vi "7HP_Get_ax_ay_az.vi"(6 "7HP Name":string, 9 "Time Trace":T1[](array[typedef]), 10 "Analysis Info cluster":T2[](array[typedef]) {"Sync Delay Time (s)" format="%.4f"; "Sd Error in Variance" format="%.2f"; "Skew_u" format="%.2f"; "% u'/U" format="%.2f"; "Sd Error in Mean" format="%.2f"; "Kurt_u" format="%.2f"; "u^4" format="%.2f"; "u^3" format="%.2f"; "U" format="%.2f"; "u^2" format="%.2f"}, 11 "Pressure Index":i32[](array[numeric])) -> (3 "ax ay az":sgl[](array[numeric]))   [LabVIEW 2018]
uses:
  Controls/Analysis_info_cluster.ctl
  Controls/Inst_type.ctl
  Controls/Instrument_Array.ctl
  Controls/Time_Trace_Cluster.ctl
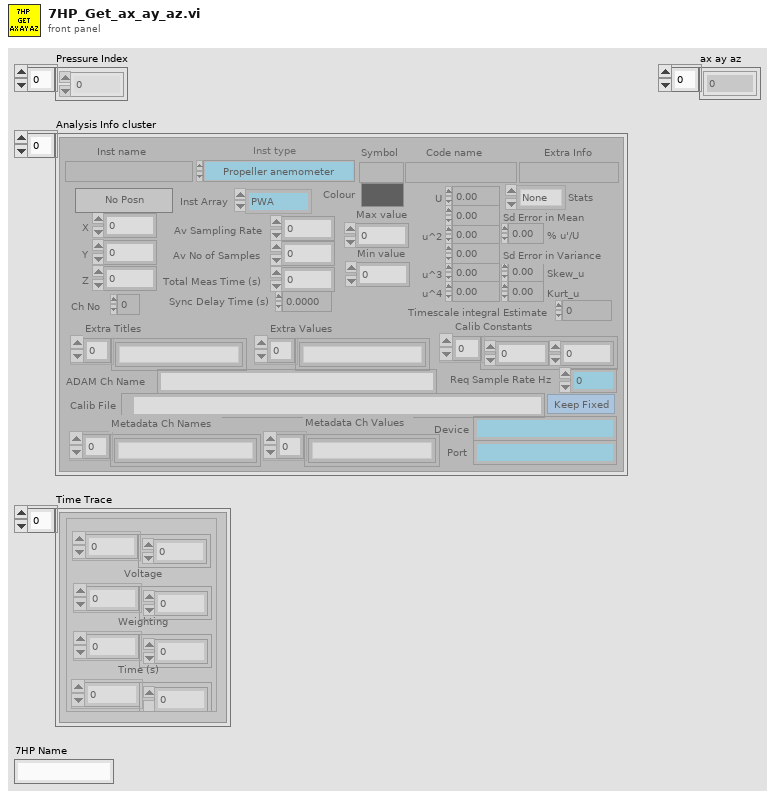
[diagram p1: front panel]
types:
  T1 = typedef "Time_Trace_Cluster.ctl" = cluster{"Weighting":dbl[], "Time (s)":dbl[], "Voltage":dbl[], "Eng Values":dbl[]}
  T2 = typedef "Analysis_info_cluster.ctl" = cluster{"Colour":u32, "Inst type":T3, "Inst name":string, "Symbol":string, "Code name":string, "Extra Info":string, "Inst Array":T4, "Extra Titles":string[], "Extra Values":string[], "U":dbl, "u^2":dbl, "u^3":dbl, "u^4":dbl, "Skew_u":dbl, "Kurt_u":dbl, "Sd Error in Mean":dbl, "% u'/U":dbl, "X":dbl, "Y":dbl, "Z":dbl, "Timescale integral Estimate":dbl, "Sd Error in Variance":dbl, "Calib File":path, "Calib Constants":dbl[], "Output Position":bool, "Stats":enum16{"None", "Basic", "Full"}, "Av Sampling Rate":dbl, "Av No of Samples":dbl, "Total Meas Time (s)":dbl, "ADAM Ch Name":string, "Max value":dbl, "Min value":dbl, "Req Sample Rate Hz":dbl, "Sync Delay Time (s)":dbl, "Ch No":i16, "Device":string, "Use Latest Calib":bool, "Port":string, "Metadata Ch Names":string[], "Metadata Ch Values":string[]}
  T3 = typedef "Inst_type.ctl" = enum16{"Propeller anemometer", "Raw voltage", "Pressure Transducer", "Pitot-static tube", "Preston tube", "Hot wire", "Cross wire 1", "Cross wire 2", "Generic Linear", "Generic Polynomial", "Generic BackPoly", "Fast FID", "Thermocouple", "Cold wire", "Pulsed Wire", "LDA Vel", "LDA Tran time", "LDA Arr time", "Microphone"}
  T4 = typedef "Instrument_Array.ctl" = enum16{"PWA", "LDA", "Analogue"}
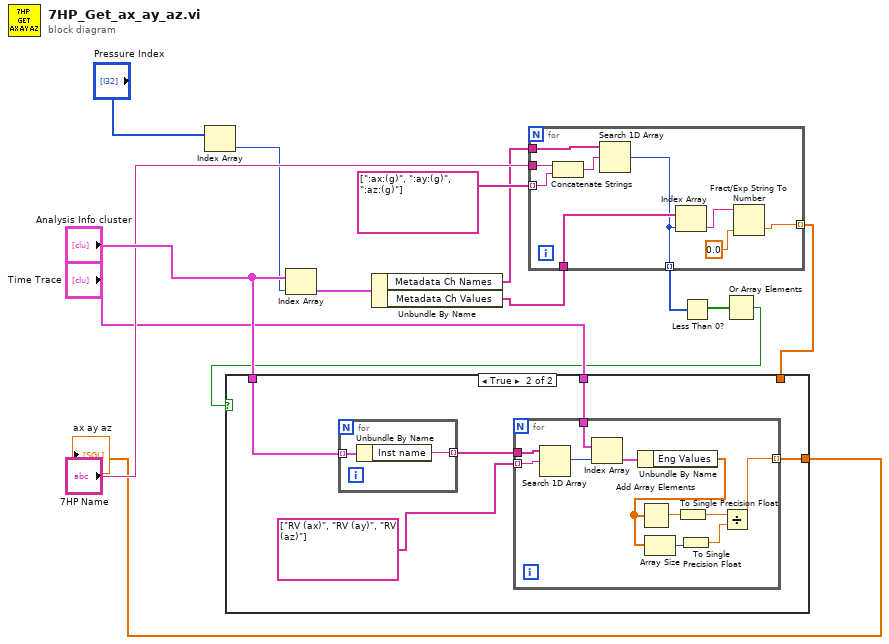
[diagram p0: block diagram]
diagram:
  n1 = Index Array(array="Pressure Index") -> (element=w2:i32)  [unwired: 1 in]
  n2 = Index Array(array="Analysis Info cluster", index=w2) -> (element=w3:T2)
  n3 = Unbundle By Name(w3) -> ("Metadata Ch Names"=w4:string[], "Metadata Ch Values"=w6:string[])
  n4 = for {
    tunnel: w4 -> [w23]
    tunnel: string[] [":ax:(g)", ":ay:(g)", ":az:(g)"] ("Metadata Ch Names") -> [w17] mode=indexing
    tunnel: w6 -> [w22]
    tunnel: [w20] -> w11 mode=indexing
    tunnel: [w18] -> w7 mode=indexing
    tunnel: "7HP Name" -> [w16]
    n5 = Concatenate Strings(w16, w17) -> (w15:string)
    n6 = Search 1D Array(1D array=w23, element=w15) -> (index of element=w18:i32)  [unwired: 1 in]
    n7 = Index Array(array=w22, index=w18) -> (element=w21:string)
    n8 = Fract/Exp String To Number(string=w21, default (0 dbl)=sgl 0.0 ("default (0 DBL)")) -> (number=w20:sgl)  [unwired: 2 in, 1 out]
  }
  n9 = Less Than 0?(x=w7) -> (x < 0?=w8:bool[])
  n10 = Or Array Elements(Boolean array=w8) -> (logical OR=w9:bool)
  n11 = case shown="True" w9 {
    tunnel: "Analysis Info cluster" -> [_ w27]
    tunnel: [w24 w26] -> w10
    tunnel: w11 -> [w24 _]
    tunnel: "Time Trace" -> [_ w25]
    frame False {
    }
    frame True {
      n12 = for {
        tunnel: w27 -> [w42] mode=indexing
        tunnel: [w41] -> w29 mode=indexing
        n13 = Unbundle By Name(w42) -> ("Inst name"=w41:string)
      }
      n14 = for {
        tunnel: w29 -> [w40]
        tunnel: string[] ["RV (ax)", "RV (ay)", "RV (az)"] ("Metadata Ch Names") -> [w39] mode=indexing
        tunnel: w25 -> [w37]
        tunnel: [w33] -> w26 mode=indexing
        n15 = Search 1D Array(1D array=w40, element=w39) -> (index of element=w38:i32)  [unwired: 1 in]
        n16 = Index Array(array=w37, index=w38) -> (element=w36:T1)
        n17 = Unbundle By Name(w36) -> ("Eng Values"=w34:dbl[])
        n18 = Add Array Elements(numeric array=w34) -> (sum=w31:dbl)
        n19 = Array Size(array=w34) -> (size(s)=w32:i32)
        n20 = To Single Precision Float(number=w31) -> (single precision float=w30:sgl)
        n21 = To Single Precision Float(number=w32) -> (single precision float=w35:sgl)
        n22 = Divide(x=w30, y=w35) -> (x/y=w33:sgl)
      }
    }
  }
  "ax ay az" <- w10
